vi "UART Write Data.vi"(7 "UART #":T1=-1, 8 "error in (no error)":errorcluster, 10 "Data":string, 11 "VisaComms in":refnum<class "VisaComms.lvclass">) -> (0 "error out":errorcluster, 3 "VisaComms out":refnum<class "VisaComms.lvclass">)   [LabVIEW 2020, in "CTI.lvlib" / "VisaComms.lvclass"]
uses:
  VisaComms.lvclass
  VisaComms.lvclass/VisaComms.ctl
  UART Number.ctl
  CTI.lvlib
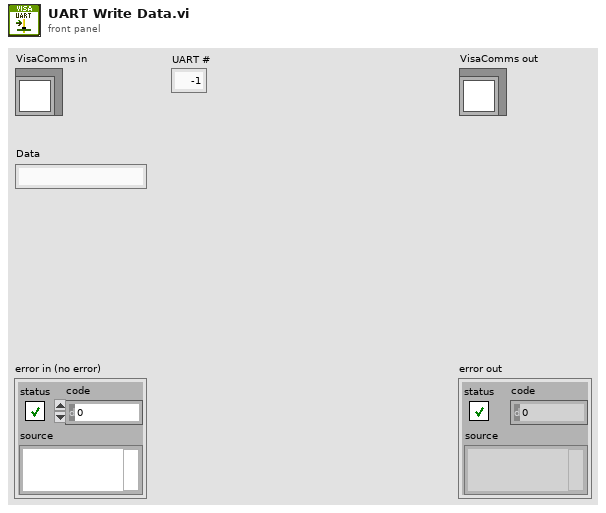
[diagram p1: front panel]
types:
  T1 = typedef "CTI.lvlib/UART Number.ctl" = i8
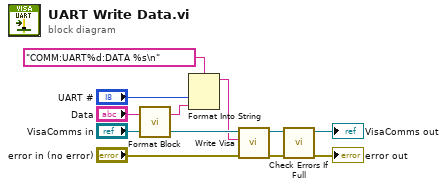
[diagram p0: block diagram]
diagram:
  n1 = call "Format Block.vi"("Data"="Data") -> ("Formatted Block"=w8:string)  [unwired: 6 in]
  n2 = Format Into String(format string="COMM:UART%d:DATA %s\n", "UART #", w8) -> (resulting string=w4:string)  [unwired: 2 in, 1 out]
  n3 = call "Write Visa.vi"("error in (no error)"="error in (no error)", "write buffer"=w4, "VisaComms in"="VisaComms in") -> ("error out"=w6:errorcluster, "VisaComms out"=w2:refnum<class "VisaComms.lvclass">)  [unwired: 6 in, 1 out]
  n4 = call "Check Errors If Full.vi"("error in (no error)"=w6, "VisaComms in"=w2) -> ("error out"=→"error out":errorcluster, "VisaComms out"=→"VisaComms out":refnum<class "VisaComms.lvclass">)  [unwired: 8 in]
